vi "Create Options Set.vi"(8 "error in (no error)":errorcluster, 11 "Options":T1[](array[typedef])) -> (0 "error out":errorcluster, 3 "Option Set out":refnum<class "Option Set.lvclass">)   [LabVIEW 2011, in "Option Parser.lvlib" / "Option Set.lvclass"]
doc: "Creates a set of options which you might expect for your application."
uses:
  Option Set.lvclass
  Option Class/Option Configuration.ctl
  Option Class/Argument Type.ctl
  Option Set.lvclass/Option Set.ctl
  Option Class/Option.lvclass
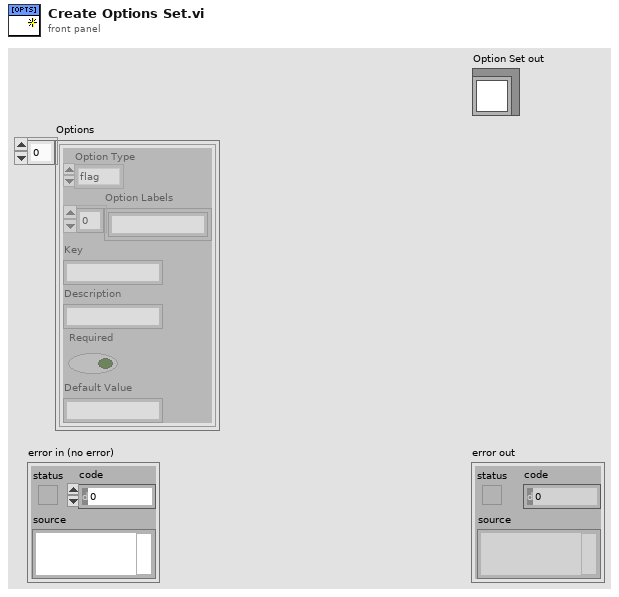
[diagram p1: front panel]
types:
  T1 = typedef "Option Parser.lvlib/Option.lvclass/Option Configuration.ctl" = cluster{"Option Type":T2, "Option Labels":string[], "Key":string, "Description":string, "Required":bool, "Default Value":string}
  T2 = typedef "Option Parser.lvlib/Option.lvclass/Argument Type.ctl" = enum16{"flag", "value"}
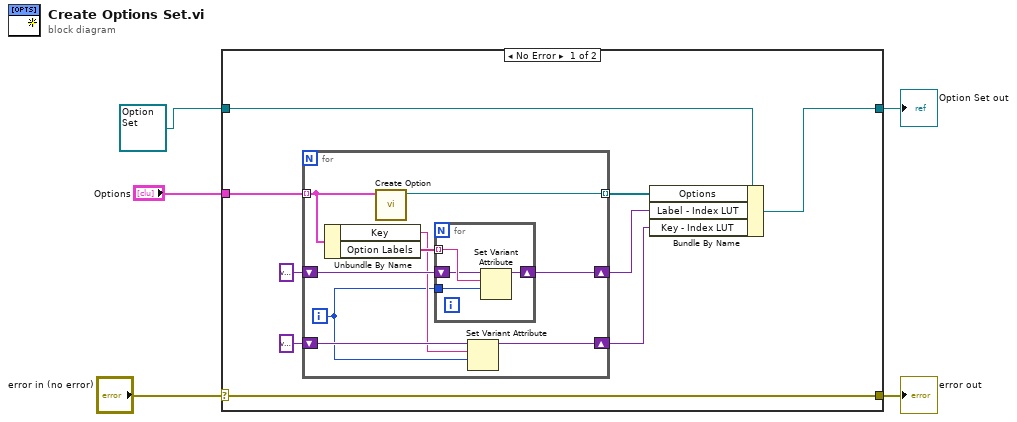
[diagram p0: block diagram]
diagram:
  n1 = case shown="No Error" "error in (no error)" {
    selector: "error in (no error)" -> [w13 w29]
    tunnel: [w13 w29] -> w4
    tunnel: [w10 w28] -> w3
    tunnel: refnum<class "Option Set.lvclass"> refnum ("Option Set in") -> [w14 w28]
    tunnel: "Options" -> [w12 _]
    frame No Error {
      n2 = for {
        tunnel: w12 -> [w23] mode=indexing
        shift-right: [w21] -> w8
        shift-left: variant -> [w20]
        tunnel: [w19] -> w9 mode=indexing
        shift-right: [w18] -> w6
        shift-left: variant -> [w17]
        i -> [w15]
        n3 = Unbundle By Name(w23) -> ("Key"=w16:string, "Option Labels"=w22:string[])
        n4 = call "Create Option.vi"("Option Config"=w23) -> ("Option out"=w19:refnum<class "Option.lvclass">)  [unwired: 9 in, 1 out]
        n5 = for {
          tunnel: w22 -> [w27] mode=indexing
          tunnel: w15 -> [w26]
          shift-right: [w25] -> w21
          shift-left: w20 -> [w24]
          n6 = Set Variant Attribute(Variant=w24, name=w27, value=w26) -> (Variant out=w25:variant)  [unwired: 1 in, 2 out]
        }
        n7 = Set Variant Attribute(Variant=w17, name=w16, value=w15) -> (Variant out=w18:variant)  [unwired: 1 in, 2 out]
      }
      n8 = Bundle By Name(cluster=w14, "Options"=w9, "Label - Index LUT"=w8, "Key - Index LUT"=w6) -> (w10:refnum<class "Option Set.lvclass">)
    }
    frame Error {
    }
  }
  "error out" <- w4
  "Option Set out" <- w3
